vi "GetDataForExcel.ReadPatientData.vi"(11 "Path":path) -> (3 "output cluster":T1)   [LabVIEW 2013, in "main.lvlib"]
uses:
  main.lvlib
  <userlib>/_OpenG.lib/file/file.llb/File Exists - Scalar__ogtk.vi
  <vilib>/Utility/file.llb/Read From Spreadsheet File (string).vi
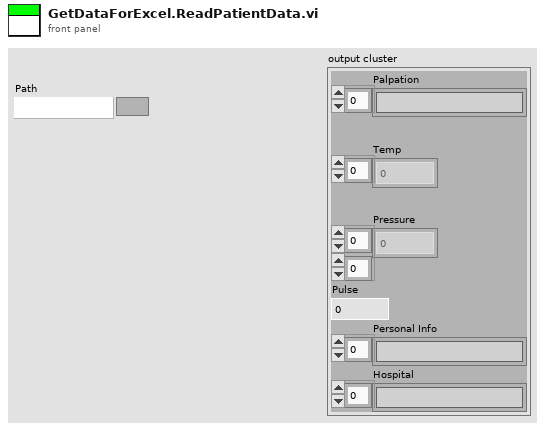
[diagram p1: front panel]
types:
  T1 = cluster{"Palpation":string[], "Temp":i32[], "Pressure":dbl[][], "Pulse":dbl, "Personal Info":string[], "Hospital":string[]}
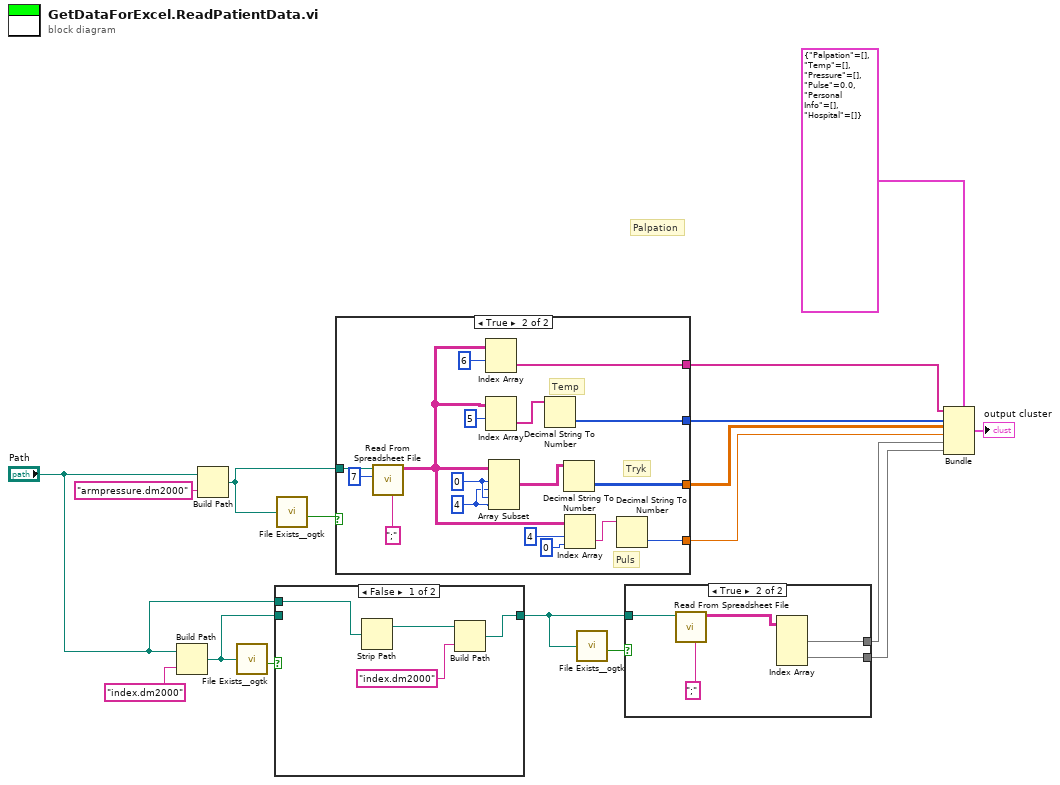
[diagram p0: block diagram]
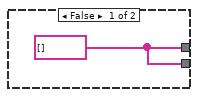
[diagram p2: hidden frame]
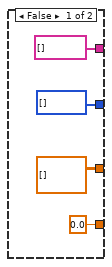
[diagram p4: hidden frame]
diagram:
  # "Palpation"
  n1 = Build Path(base path="Path", name or relative path="index.dm2000") -> (appended path=w11:path)
  n2 = Build Path(base path="Path", name or relative path="armpressure.dm2000") -> (appended path=w8:path)
  n3 = call-poly <userlib>:"File Exists__ogtk.vi"("file path"=w11) -> ("exists"=w10:bool)  [unwired: 6 in, 1 out]
  n4 = case shown="False" w10 {
    tunnel: "Path" -> [w20 _]
    tunnel: [w21 w22] -> w12
    tunnel: w11 -> [_ w22]
    frame False {
      n5 = Strip Path(path=w20) -> (stripped path=w19:path)  [unwired: 1 out]
      n6 = Build Path(base path=w19, name or relative path="index.dm2000") -> (appended path=w21:path)
    }
    frame True {
    }
  }
  n7 = call-poly <userlib>:"File Exists__ogtk.vi"("file path"=w8) -> ("exists"=w9:bool)  [unwired: 6 in, 1 out]
  n8 = case shown="True" w9 {
    tunnel: w8 -> [_ w37]
    tunnel: [dbl[][] [] w35] -> w14
    tunnel: [0.0 w33] -> w15
    tunnel: [string[] [] w28] -> w2
    tunnel: [i32[] [] w27] -> w1
    frame False {
    }
    frame True {
      w38 = 4 ("length")
      w39 = 0 ("index")
      # "Tryk"
      # "Puls"
      # "Temp"
      n9 = call-poly <vilib>:"Read From Spreadsheet File.vi"("delimiter (\\t)"=";" ("delimiter (\\t)"), "number of rows (all:-1)"=7, "file path (dialog if empty)"=w37) -> ("all rows"=w29:string[][])  [unwired: 4 in, 4 out]
      n10 = Index Array(array=w29, index (row)=6) -> (element=w28:string[])  [unwired: 1 in]
      n11 = Index Array(array=w29, index (row)=5 ("index")) -> (element=w31:string[])  [unwired: 1 in]
      n12 = Array Subset(array=w29, index (row)=w39, length (row)=w38, index (col)=w39, length (col)=w38) -> (w36:string[][])
      n13 = Decimal String To Number(string=w31) -> (number=w27:i32[])  [unwired: 2 in, 1 out]
      n14 = Decimal String To Number(string=w36) -> (number=w35:i32[][])  [unwired: 2 in, 1 out]
      n15 = Index Array(array=w29, index (row)=4, index (col)=0 ("disabled index (col)")) -> (element=w34:string)
      n16 = Decimal String To Number(string=w34) -> (number=w33:i32)  [unwired: 2 in, 1 out]
    }
  }
  n17 = call-poly <userlib>:"File Exists__ogtk.vi"("file path"=w12) -> ("exists"=w13:bool)  [unwired: 6 in, 1 out]
  n18 = case shown="True" w13 {
    tunnel: [w44 w48] -> w16
    tunnel: [w44 w46] -> w17
    tunnel: w12 -> [_ w45]
    frame False {
      w44 = string[] [] ("all rows")
    }
    frame True {
      n19 = call-poly <vilib>:"Read From Spreadsheet File.vi"("delimiter (\\t)"=";" ("delimiter (\\t)"), "file path (dialog if empty)"=w45) -> ("all rows"=w47:string[][])  [unwired: 5 in, 4 out]
      n20 = Index Array(array=w47) -> (element #1=w48:string[], element #2=w46:string[])  [unwired: 4 in]
    }
  }
  n21 = Bundle(cluster=T1 {"Palpation"=[], "Temp"=[], "Pressure"=[], "Pulse"=0.0, "Personal Info"=[], "Hospital"=[]} ("output cluster"), "Palpation"=w2, "Temp"=w1, "Pressure"=w14, "Pulse"=w15, "Personal Info"=w16, "Hospital"=w17) -> (→"output cluster":T1)
